vi "startStartStopFGV.vi"(9 "stop":bool, 10 "start":bool, 11 "Enum":T1) -> (1 "stop":bool, 2 "start":bool)   [LabVIEW 2017]
uses:
  TypeDefs/starFGVControl.ctl
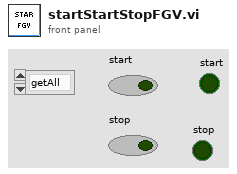
[diagram p1: front panel]
types:
  T1 = typedef "starFGVControl.ctl" = enum16{"getAll", "setStop", "setStart"}
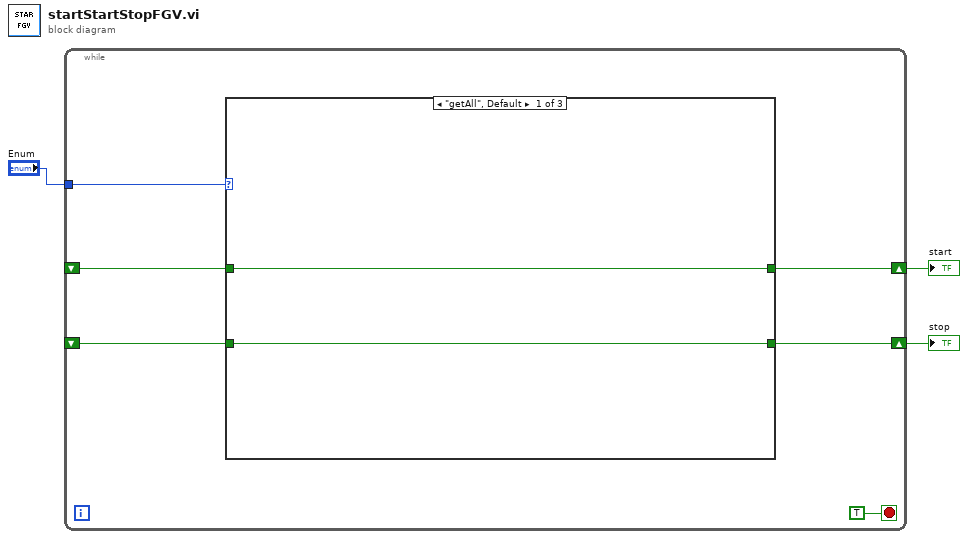
[diagram p0: block diagram]
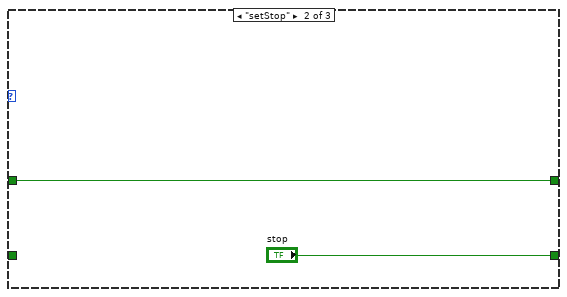
[diagram p2: hidden frame]
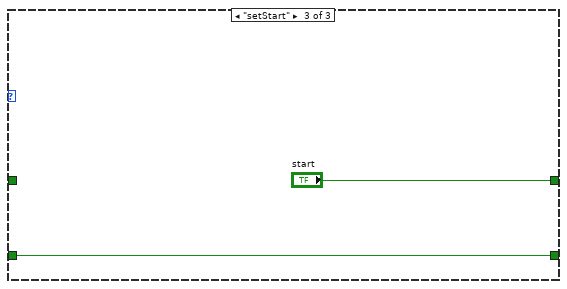
[diagram p3: hidden frame]
diagram:
  n1 = while {
    tunnel: "Enum" -> [w9]
    shift-right: [w7] -> w2
    shift-left: _ -> [w4]
    shift-right: [w6] -> w1
    shift-left: _ -> [w5]
    stop <- TRUE stop-if-true
    n2 = case shown="\"getAll\", Default" w9 {
      tunnel: [w10 "stop" w15] -> w7
      tunnel: [w11 w12 "start"] -> w6
      tunnel: w5 -> [w11 w12 _]
      tunnel: w4 -> [w10 _ w15]
      frame "getAll", Default {
      }
      frame "setStop" {
      }
      frame "setStart" {
      }
    }
  }
  "stop" <- w2
  "start" <- w1
